vi "Puzzle 4-1.vi"() -> ()   [LabVIEW 2022 SP3]
panel:
  out "sum":i32
  in  "delimited string":string
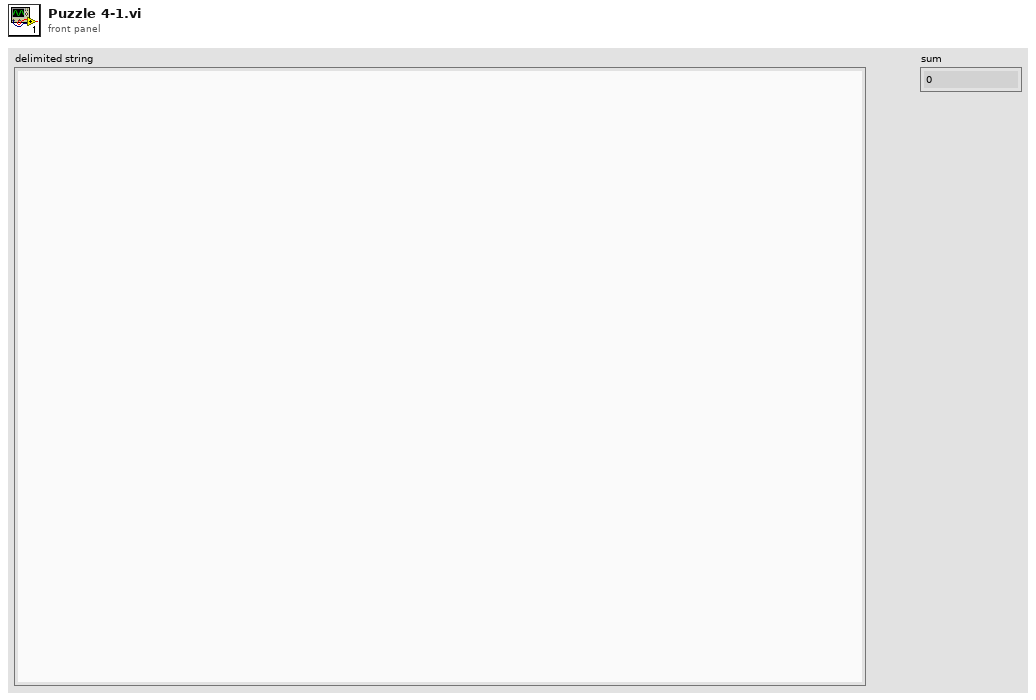
[diagram p1: front panel]
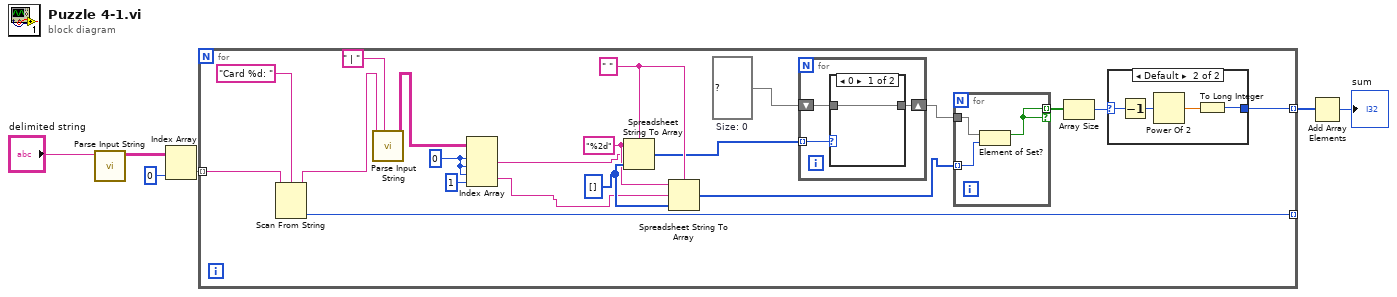
[diagram p0: block diagram]
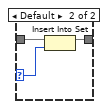
[diagram p3: hidden frame]
diagram:
  n1 = call "Parse Input String.vi"("delimited string"="delimited string") -> ("parsed string"=w5:string[][])  [unwired: 10 in]
  n2 = Index Array(array=w5, index (col)=0 ("disabled index (col)")) -> (element=w3:string[])  [unwired: 1 in]
  n3 = for {
    tunnel: w3 -> [w26] mode=indexing
    tunnel: [w24] -> _ mode=indexing
    tunnel: [w7] -> w2 mode=indexing
    w12 = set{i32} {}  # Size: 0
    w19 = i32[] [] ("array type (2D Dbl)")
    w18 = "%2d" ("format string")
    w20 = " " ("delimiter (Tab)")
    w17 = 0 ("disabled index (col)")
    n4 = Scan From String(format string="Card %d: " ("delimiter (Tab)"), input string=w26) -> (remaining string=w23:string, output 1=w24:i32)  [unwired: 3 in, 2 out]
    n5 = call "Parse Input String.vi"("delimiter (Tab)"=" | ", "delimited string"=w23) -> ("parsed string"=w21:string[][])  [unwired: 9 in]
    n6 = Index Array(array=w21, index (row) #1=w17, index (col) #1=w17, index (row) #2=w17, index (col) #2=1 ("disabled index (col)")) -> (element #1=w15:string, element #2=w14:string)
    n7 = Spreadsheet String To Array(delimiter (Tab)=w20, format string=w18, spreadsheet string=w15, array type (2D Dbl)=w19) -> (array=w13:i32[])
    n8 = Spreadsheet String To Array(delimiter (Tab)=w20, format string=w18, spreadsheet string=w14, array type (2D Dbl)=w19) -> (array=w11:i32[])
    n9 = for {
      tunnel: w13 -> [w37] mode=indexing
      shift-right: [w36] -> w10
      shift-left: w12 -> [w35]
      n10 = case shown="0" w37 {
        selector: w37 -> [_ w41]
        tunnel: [w38 w40] -> w36
        tunnel: w35 -> [w38 w39]
        frame 0 {
        }
        frame Default {
          n11 = Insert Into Set(10:w41, 11:w39) -> (3:w40:set{i32})  [unwired: 1 out]
        }
      }
    }
    n12 = for {
      tunnel: w11 -> [w33] mode=indexing
      tunnel: w10 -> [w34]
      tunnel: [w32] -> w9 mode=indexing if=w32
      n13 = Element of Set?(10:w33, 11:w34) -> (3:w32:bool)
    }
    n14 = Array Size(array=w9) -> (size(s)=w8:i32)
    n15 = case shown="Default" w8 {
      selector: w8 -> [w27 w31]
      tunnel: [w27 w29] -> w7
      frame 0 {
      }
      frame Default {
        n16 = Decrement(x=w31) -> (x-1=w30:i32)
        n17 = Power Of 2(x=w30) -> (2^x=w28:dbl)
        n18 = To Long Integer(number=w28) -> (32bit integer=w29:i32)
      }
    }
  }
  n19 = Add Array Elements(numeric array=w2) -> (sum=→"sum":i32)
